vi "Finish Command.vi"(8 "error in (no error)":errorcluster, 11 "Command in":refnum<class "Command State Actor.lvclass">) -> (0 "error out":errorcluster, 3 "Command out":refnum<class "Command State Actor.lvclass">)   [LabVIEW 2013, in "Command State Actor.lvlib" / "Command State Actor.lvclass"]
uses:
  Command State Actor.lvclass
  Command States.ctl
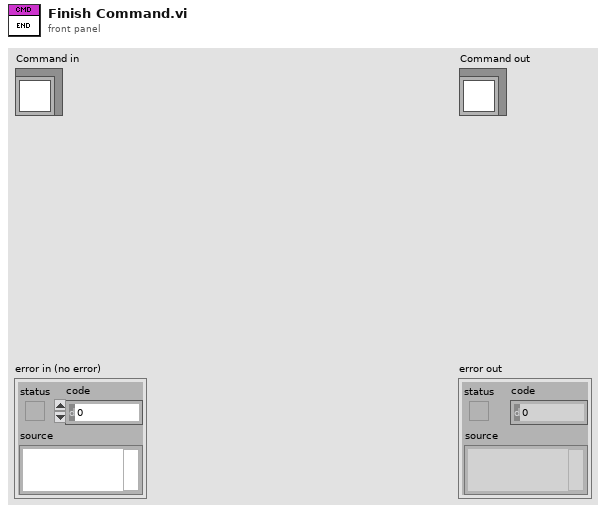
[diagram p1: front panel]
types:
  T1 = typedef "Command State Actor.lvlib/Command State Actor.lvclass/Command States.ctl" = enum16{"NotStarted", "Starting", "Started", "Executing", "Completing", "Completed", "Stopping", "Stopped"}
  T2 = typedef "Command State Actor.lvlib/Command State Actor.lvclass/Command Status.ctl" = cluster{"CurrentCommandState":T1, "Command Name":string, "Current State Status":T3, "Command Start Time":timestamp, "Command End Time":timestamp, "Previous State Status":T3}
  T3 = typedef "Command Actor.lvlib/Command States.lvclass/State Status.ctl" = cluster{"State Name":string, "State Entry Time":timestamp, "State Exit Time":timestamp}
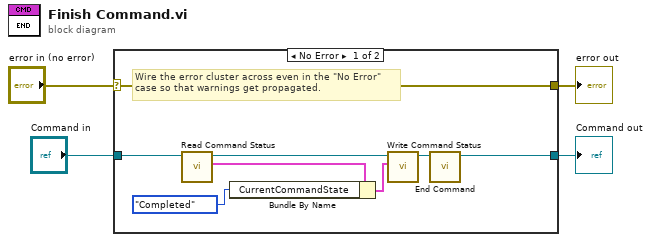
[diagram p0: block diagram]
diagram:
  n1 = case shown="No Error" "error in (no error)" {
    selector: "error in (no error)" -> [w12 w14]
    tunnel: [w12 w14] -> w3
    tunnel: [w8 w13] -> w1
    tunnel: "Command in" -> [w11 w13]
    frame No Error {
      # "Wire the error cluster across even in the \"No Error\"\ncase so that warnings get propagated."
      n2 = call-dynamic "Read Command Status.vi"("Command in"=w11) -> ("Command Status"=w7:T2, "Command out"=w10:refnum<class "Command State Actor.lvclass">)  [unwired: 8 in, 1 out]
      n3 = Bundle By Name(cluster=w7, "CurrentCommandState"=Command_States."Completed") -> (w6:T2)
      n4 = call-dynamic "Write Command Status.vi"("Command Status"=w6, "Command in"=w10) -> ("Command out"=w9:refnum<class "Command State Actor.lvclass">)  [unwired: 8 in, 1 out]
      n5 = call-dynamic "End Command.vi"("Command in"=w9) -> ("Command out"=w8:refnum<class "Command State Actor.lvclass">)  [unwired: 9 in, 1 out]
    }
    frame Error {
    }
  }
  "error out" <- w3
  "Command out" <- w1
